vi "LabFrog.vi"() -> ()   [LabVIEW 2014]
uses:
  <vilib>/regexp/Match Regular Expression.xnode
panel:
  out "filenames":string[](array[string])
  out "Frog values":string[](array[string])
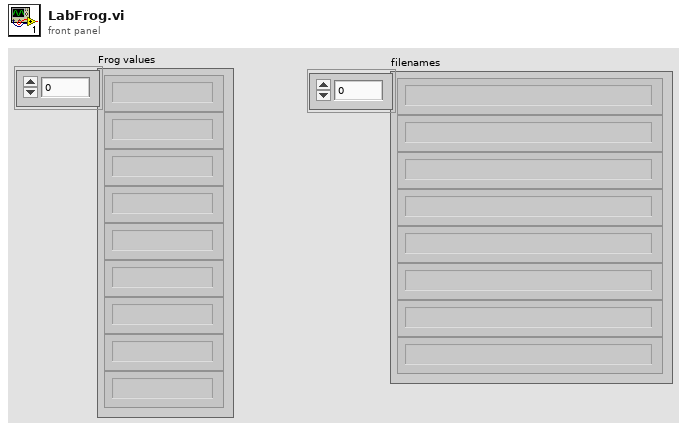
[diagram p1: front panel]
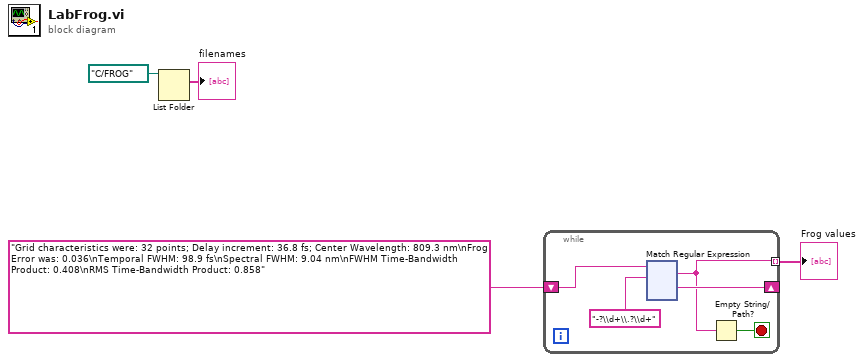
[diagram p0: block diagram]
diagram:
  n1 = List Folder(path=path "C:/FROG") -> (filenames=→"filenames":string[])  [unwired: 3 in, 3 out]
  n2 = while {
    shift-right: [w7] -> _
    shift-left: "Grid characteristics were: 32 points; Delay increment: 36.8 fs; Center Wavelength: 809.3 nm\nFrog Error was: 0.036\nTemporal FWHM: 98.9 fs\nSpectral FWHM: 9.04 nm\nFWHM Time-Bandwidth Product: 0.408\nRMS Time-Bandwidth Product: 0.858" -> [w9]
    tunnel: [w6] -> w4 mode=indexing
    stop <- w5 stop-if-true
    n3 = xnode "Match Regular Expression"("input string"=w9, "regular expression"="-?\\d+\\.?\\d+") -> ("whole match"=w6:string, "after match"=w7:string)  [unwired: 4 in, 3 out]
    n4 = Empty String/Path?(string/path=w6) -> (empty?=w5:bool)
  }
  "Frog values" <- w4
